vi "scale sticks.vi"(4 "Low Speed":dbl, 5 "Slow Mode":bool, 6 "Normal Speed":dbl, 7 "Fast Mode":bool, 8 "High Speed":dbl, 9 "Z":dbl, 10 "Y":dbl, 11 "X":dbl) -> (1 "Z Out":dbl, 2 "Y Out":dbl, 3 "X Out":dbl)   [LabVIEW 2016]
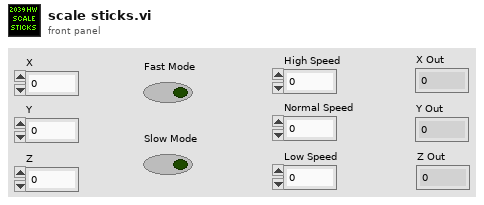
[diagram p1: front panel]
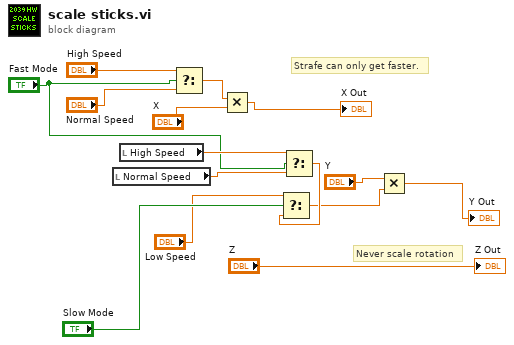
[diagram p0: block diagram]
diagram:
  # "Never scale rotation"
  # "Strafe can only get faster."
  n1 = local read "Normal Speed"() -> (w8:dbl)
  n2 = local read "High Speed"() -> (w9:dbl)
  n3 = Select(t="High Speed", s="Fast Mode", f="Normal Speed") -> (s? t:f=w13:dbl)
  n4 = Multiply(x=w13, y="X") -> (x*y=→"X Out":dbl)
  n5 = Select(t=w9, s="Fast Mode", f=w8) -> (s? t:f=w4:dbl)
  n6 = Select(t="Low Speed", s="Slow Mode", f=w4) -> (s? t:f=w2:dbl)
  n7 = Multiply(x="Y", y=w2) -> (x*y=→"Y Out":dbl)
  "Z Out" <- "Z"
